vi "Main.vi"   [LabVIEW 2011]
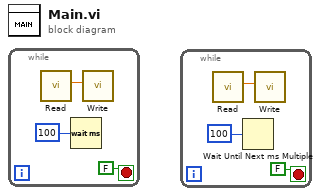
[diagram p0: block diagram]
diagram:
  n1 = while {
    stop <- FALSE stop-if-true
    n2 = call "Read.vi"() -> ("Numeric"=w2:dbl)  [unwired: 11 in]
    n3 = Wait (ms)(milliseconds to wait=u32 100) -> ()  [unwired: 1 out]
    n4 = call "Write.vi"("Numeric"=w2) -> ()  [unwired: 11 in]
  }
  n5 = while {
    stop <- FALSE stop-if-true
    n6 = call "Read.vi"() -> ("Numeric"=w5:dbl)  [unwired: 11 in]
    n7 = Wait Until Next ms Multiple(millisecond multiple=u32 100) -> ()  [unwired: 1 out]
    n8 = call "Write.vi"("Numeric"=w5) -> ()  [unwired: 11 in]
  }
